vi "fgvTcpQueueTx.vi"(8 "Error In":errorcluster caption="에러 입력", 9 "Urgent":bool, 10 "Write":string, 11 "Function":T1) -> (0 "Error Out":errorcluster caption="에러 출력", 2 "Read":string, 3 "Count":i32)   [LabVIEW 2018]
uses:
  control/enumFgvFunction.ctl
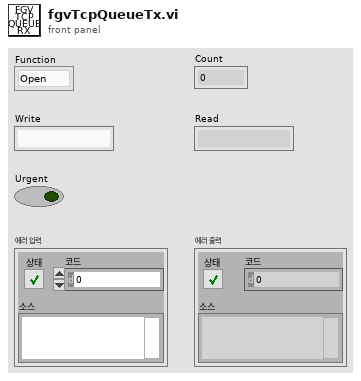
[diagram p1: front panel]
types:
  T1 = typedef "enumFgvFunction.ctl" = enum16{"Open", "Read", "Check", "Write", "Close"}
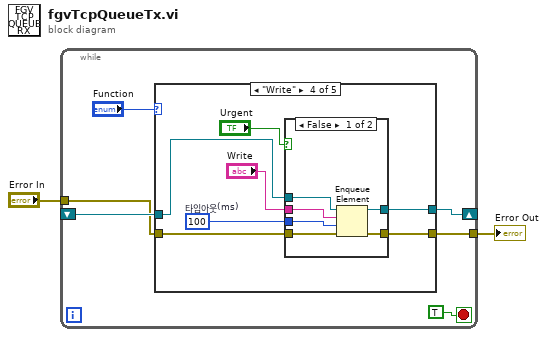
[diagram p0: block diagram]
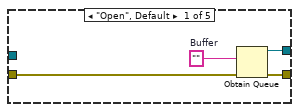
[diagram p2: hidden frame]
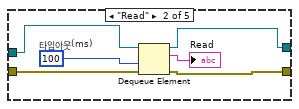
[diagram p3: hidden frame]
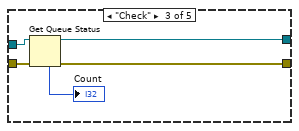
[diagram p4: hidden frame]
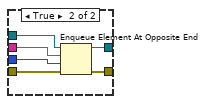
[diagram p5: hidden frame]
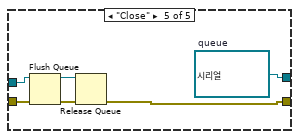
[diagram p6: hidden frame]
diagram:
  n1 = while {
    shift-right: [w6] -> _
    shift-left: _ -> [w7]
    tunnel: "Error In" -> [w5]
    tunnel: [w4] -> w1
    stop <- TRUE stop-if-true
    n2 = case shown="\"Write\"" "Function" {
      tunnel: w7 -> [_ w18 w23 w30 w48]
      tunnel: [w12 w17 w22 w29 w46] -> w6
      tunnel: w5 -> [w9 w15 w20 w27 w45]
      tunnel: [w10 w14 w19 w26 w43] -> w4
      frame "Open", Default {
        w11 = ""  # Buffer
        n3 = Obtain Queue(element data type=w11, error in (no error)=w9) -> (queue out=w12:refnum<queue>, error out=w10:errorcluster)  [unwired: 3 in, 1 out]
      }
      frame "Read" {
        w13 = 100  # 타임아웃(ms)
        n4 = Dequeue Element(queue=w18, timeout in ms (-1)=w13, error in (no error)=w15) -> (queue out=w17:refnum<queue>, element=→"Read":string, error out=w14:errorcluster)  [unwired: 1 out]
      }
      frame "Check" {
        n5 = Get Queue Status(queue=w23, error in (no error)=w20) -> (queue out=w22:refnum<queue>, error out=w19:errorcluster, # elements in queue=→"Count":i32)  [unwired: 1 in, 5 out]
      }
      frame "Write" {
        w25 = 100  # 타임아웃(ms)
        n6 = case shown="False" "Urgent" {
          tunnel: w30 -> [w36 w42]
          tunnel: [w35 w41] -> w29
          tunnel: "Write" -> [w34 w37]
          tunnel: w27 -> [w33 w39]
          tunnel: [w32 w40] -> w26
          tunnel: w25 -> [w31 w38]
          frame False {
            n7 = Enqueue Element(queue=w36, element=w34, timeout in ms (-1)=w31, error in (no error)=w33) -> (queue out=w35:refnum<queue>, error out=w32:errorcluster)  [unwired: 1 out]
          }
          frame True {
            n8 = Enqueue Element At Opposite End(queue=w42, element=w37, timeout in ms (-1)=w38, error in (no error)=w39) -> (queue out=w41:refnum<queue>, error out=w40:errorcluster)  [unwired: 1 out]
          }
        }
      }
      frame "Close" {
        w46 = refnum<queue> refnum  # queue
        n9 = Flush Queue(queue=w48, error in (no error)=w45) -> (queue out=w47:refnum<queue>, error out=w44:errorcluster)  [unwired: 1 out]
        n10 = Release Queue(queue=w47, error in (no error)=w44) -> (error out=w43:errorcluster)  [unwired: 1 in, 2 out]
      }
    }
  }
  "Error Out" <- w1
